vi "get_path_from_root_folder.vi"(11 "Path":path) -> (1 "Number of Files":i32, 3 "Array":path[](array[path]))   [LabVIEW 2020]
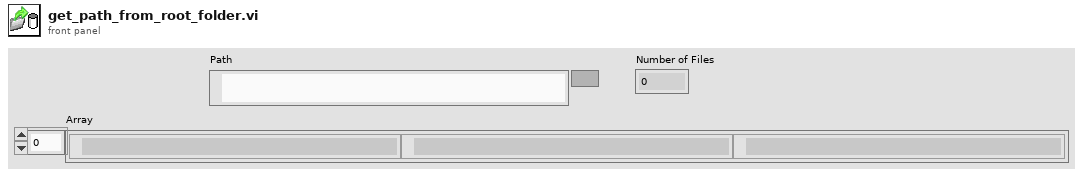
[diagram p1: front panel]
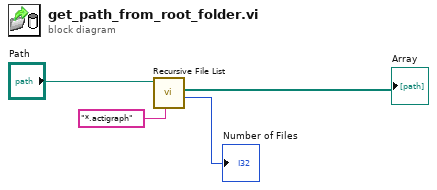
[diagram p0: block diagram]
diagram:
  n1 = call <vilib>:"Recursive File List.vi"("pattern"="*.actigraph", "Folder Path"="Path") -> ("Number of Files"=→"Number of Files":i32, "All Files in Dir"=→"Array":path[])  [unwired: 5 in, 3 out]
